vi "Draw.vi"(8 "Error In":errorcluster, 9 "Coordinants":cluster{"X":i16, "Y":i16}, 10 "2D Picture In":picture, 11 "Square in":refnum<class "Square.lvclass">) -> (0 "Error Out":errorcluster, 2 "2D Picture Out":picture, 3 "Square out":refnum<class "Square.lvclass">)   [LabVIEW 2021, in "Square.lvclass"]
doc: "Draw a square on 2D picture.\nCoordinates is positison of left upper corner of this figure."
uses:
  Square.lvclass
  Rectangle/Rectangle.lvclass
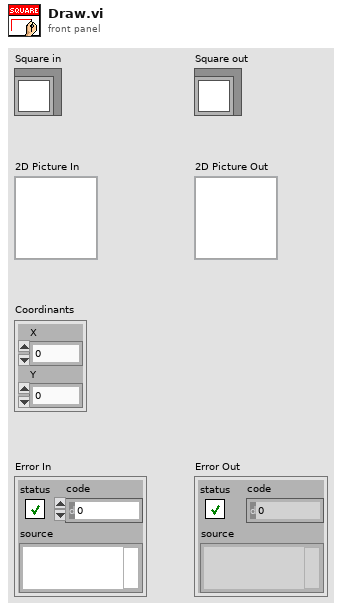
[diagram p1: front panel]
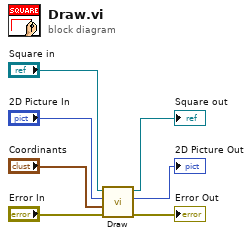
[diagram p0: block diagram]
diagram:
  n1 = call-parent "Draw.vi"("Error In"="Error In", "Coordinants"="Coordinants", "2D Picture In"="2D Picture In", "Rectangle in"="Square in") -> ("Error Out"=→"Error Out":errorcluster, "2D Picture Out"=→"2D Picture Out":picture, "Rectangle out"=→"Square out":refnum<class "Square.lvclass">)  [unwired: 5 in]
